vi "ConvertDNetCommandRegister.vi"(1 "CommandRegisterBit Array":bool[](array[boolean])) -> ()   [LabVIEW 2011]
uses:
  Controls/DNet CommandRegister Cluster.ctl
  GlobalVariables.vi
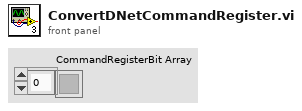
[diagram p1: front panel]
types:
  T1 = typedef "DNet CommandRegister Cluster.ctl" = cluster{"Run":bool, "Fault":bool, "DisableNetowrk":bool, "HaltScanner":bool, "Reset":bool}
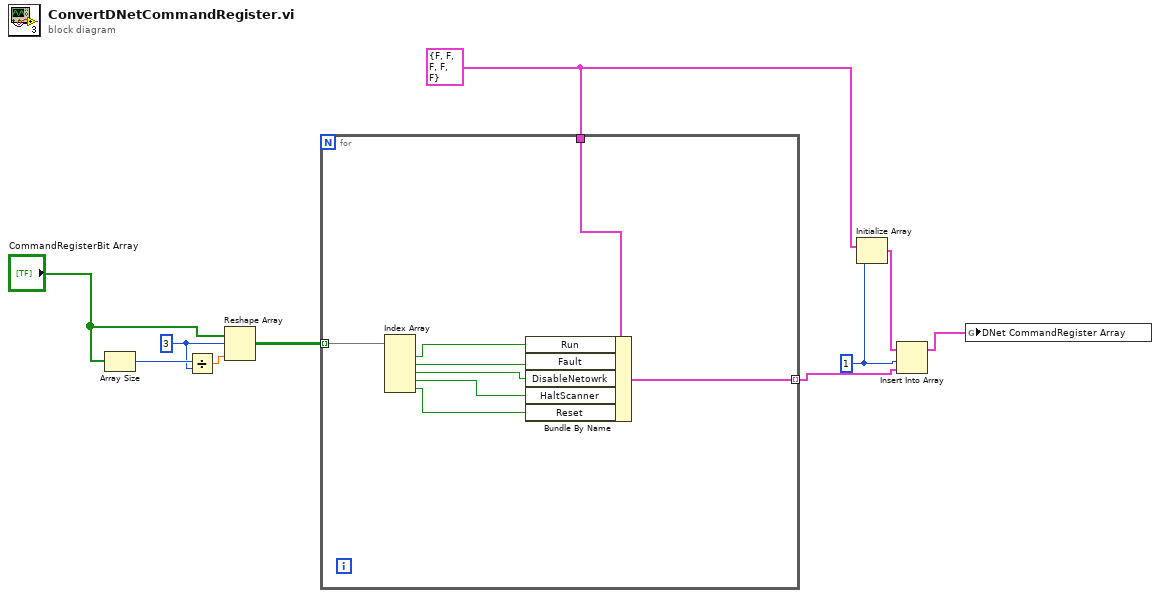
[diagram p0: block diagram]
diagram:
  w4 = 1 ("index")
  w1 = T1 {"Run"=FALSE, "Fault"=FALSE, "DisableNetowrk"=FALSE, "HaltScanner"=FALSE, "Reset"=FALSE} ("DNet CommandRegister Cluster")
  w8 = 3 ("dimension size")
  n1 = Array Size(array="CommandRegisterBit Array") -> (size(s)=w10:i32)
  n2 = Divide(x=w10, y=w8) -> (x/y=w9:dbl)
  n3 = Reshape Array("CommandRegisterBit Array", w8, w9) -> (w6:bool[][])
  n4 = for {
    tunnel: w6 -> [w18] mode=indexing
    tunnel: w1 -> [w17]
    tunnel: [w11] -> w3 mode=indexing
    n5 = Index Array(array=w18) -> (element #1=w16:bool, element #2=w15:bool, element #3=w14:bool, element #4=w13:bool, element #5=w12:bool)  [unwired: 5 in]
    n6 = Bundle By Name(cluster=w17, "Run"=w16, "Fault"=w15, "DisableNetowrk"=w14, "HaltScanner"=w13, "Reset"=w12) -> (w11:T1)
  }
  n7 = Initialize Array(w1, w4) -> (w5:T1[])
  n8 = Insert Into Array(array=w5, index=w4, new element=w3) -> (w2:T1[])
  n9 = global write "GlobalVariables.vi" "DNet CommandRegister Array"(w2) -> ()
